vi "Poisson Moments.vi"(10 "lambda":dbl=1.0) -> (0 "error":i32, 2 "variance":dbl=1.0, 3 "mean":dbl=1.0)   [LabVIEW 2018, in "NI_Gmath.lvlib"]
doc: "Returns the expected mean and variance of the random variate X, where X describes the selected distribution type. You must manually select the polymorphic instance to use."
uses:
  NI_Gmath.lvlib
  st_error_code.ctl
panel:
  # "Poisson Moments"
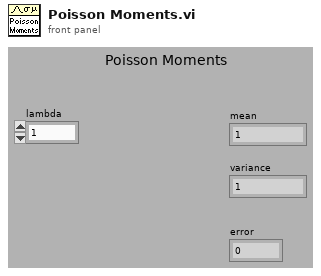
[diagram p1: front panel]
types:
  T1 = typedef "NI_Gmath.lvlib/st_error_code.ctl" = i32
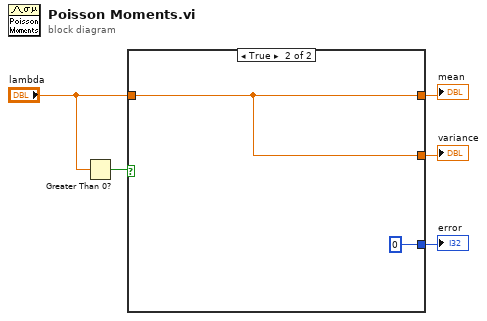
[diagram p0: block diagram]
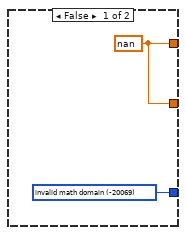
[diagram p2: hidden frame]
diagram:
  n1 = Greater Than 0?(x="lambda") -> (x > 0?=w5:bool)
  n2 = case shown="True" w5 {
    tunnel: [w6 w8] -> w2
    tunnel: [w7 0 ("error")] -> w1
    tunnel: "lambda" -> [_ w8]
    tunnel: [w6 w8] -> w3
    frame False {
      w7 = T1 -20069 items=["invalid math domain"=-20069, "Fourier interpolation size m >= n"=-20070, "empty array"=-20003] ("stat interp error code")
      w6 = nan
    }
    frame True {
    }
  }
  "error" <- w1
  "mean" <- w2
  "variance" <- w3
